vi "_API_BINANCE_GET_AccountStatus.vi"(0 "BinanceAPI in":refnum<class "BinanceAPI_.lvclass">, 11 "error in (no error)":errorcluster) -> (4 "BinanceAPI out":refnum<class "BinanceAPI_.lvclass">, 6 "Account ok?":bool, 14 "Dane":string, 15 "error out":errorcluster)   [LabVIEW 2022 SP3, in "BinanceAPI_.lvclass"]
doc: "https://binance-docs.github.io/apidocs/spot/en/#account-status-user_data"
uses:
  BinanceAPI_.lvclass
  BinanceAPI_.lvclass/BinanceAPI_.ctl
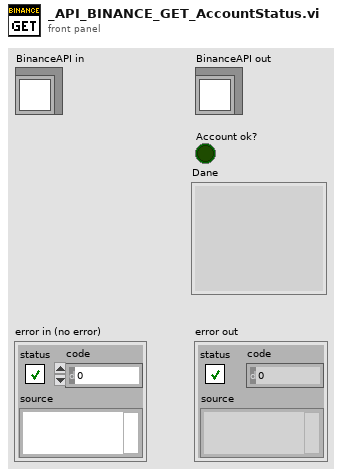
[diagram p1: front panel]
types:
  T1 = enum16{"SPOT", "USDT_FUTURES", "COIN_FUTURES", "VANILLA"}
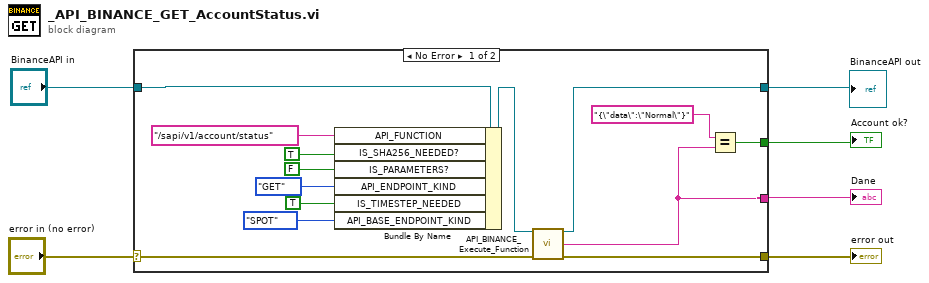
[diagram p0: block diagram]
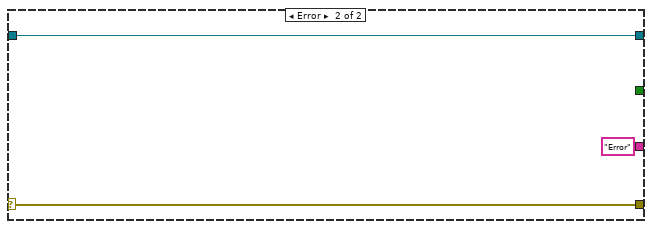
[diagram p2: hidden frame]
diagram:
  n1 = case shown="No Error" "error in (no error)" {
    selector: "error in (no error)" -> [w12 w23]
    tunnel: [w11 w23] -> w5
    tunnel: [w13 w22] -> w1
    tunnel: "BinanceAPI in" -> [w17 w22]
    tunnel: [w8 "Error" ("Dane")] -> w4
    tunnel: [w7 _] -> w3
    frame No Error {
      n2 = Bundle By Name(cluster=w17, "API_FUNCTION"="/sapi/v1/account/status", "IS_SHA256_NEEDED?"=TRUE, "IS_PARAMETERS?"=FALSE, "API_ENDPOINT_KIND"=enum16{"POST", "DELETE", "GET", "PUT"}."GET", "IS_TIMESTEP_NEEDED"=TRUE, "API_BASE_ENDPOINT_KIND"=T1."SPOT") -> (w14:refnum<class "BinanceAPI_.lvclass">)
      n3 = call "API_BINANCE_Execute_Function.vi"("BinanceAPI in"=w14, "error in (no error)"=w12) -> ("BinanceAPI out"=w13:refnum<class "BinanceAPI_.lvclass">, "Body"=w8:string, "error out"=w11:errorcluster)  [unwired: 9 in, 2 out]
      n4 = Equal?(x="{\"data\":\"Normal\"}" ("Body"), y=w8) -> (x = y?=w7:bool)
    }
    frame Error {
    }
  }
  "error out" <- w5
  "Dane" <- w4
  "Account ok?" <- w3
  "BinanceAPI out" <- w1
